vi "Sort group type.vi"(8 "error in (no error)":errorcluster, 11 "Paged groups":string[][](array[string])) -> (0 "error out":errorcluster, 2 "Group Stanards":string[][](array[string]), 3 "Group Unknowns":string[][](array[string]))   [LabVIEW 2016]
doc: "This takes the group data and sorts it into 2d array or either standards or unknowns."
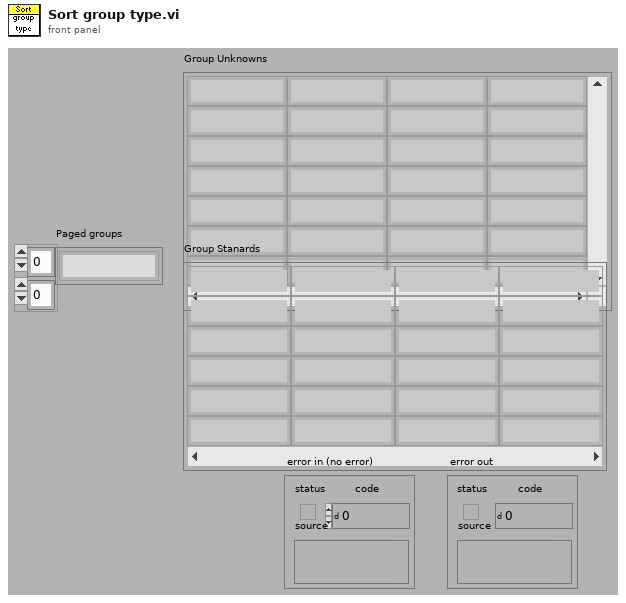
[diagram p1: front panel]
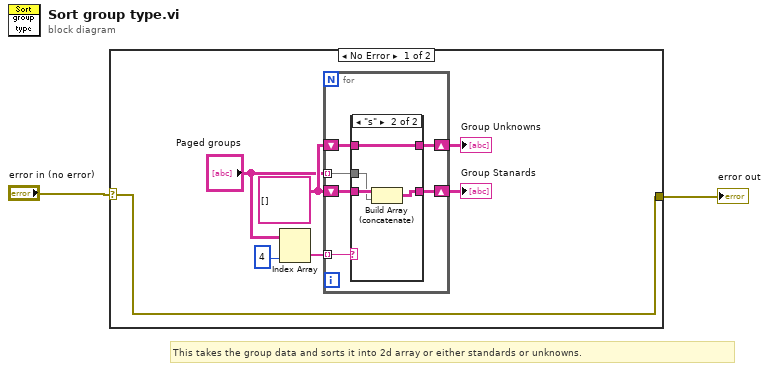
[diagram p0: block diagram]
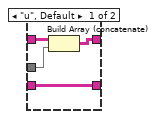
[diagram p2: hidden frame]
diagram:
  # "This takes the group data and sorts it into 2d array or either standards or unknowns."
  n1 = case shown="No Error" "error in (no error)" {
    selector: "error in (no error)" -> [w3 w24]
    tunnel: [w3 w24] -> w1
    frame No Error {
      w7 = string[][] []
      n2 = Index Array(array="Paged groups", index (col)=4 ("disabled index (col)")) -> (element=w5:string[])  [unwired: 1 in]
      n3 = for {
        tunnel: w5 -> [w15] mode=indexing
        tunnel: "Paged groups" -> [w14] mode=indexing
        shift-right: [w13] -> w8
        shift-left: w7 -> [w12]
        shift-right: [w11] -> w9
        shift-left: w7 -> [w10]
        n4 = case shown="\"s\"" w15 {
          tunnel: w14 -> [w19 w20]
          tunnel: [w18 w23] -> w13
          tunnel: w12 -> [w17 w23]
          tunnel: [w16 w22] -> w11
          tunnel: w10 -> [w16 w21]
          frame "u", Default {
            n5 = Build Array (concatenate)(w17, w19) -> (w18:string[][])
          }
          frame "s" {
            n6 = Build Array (concatenate)(w21, w20) -> (w22:string[][])
          }
        }
      }
      "Group Unknowns" <- w8
      "Group Stanards" <- w9
    }
    frame Error {
    }
  }
  "error out" <- w1
